vi "Read Port.vi"(8 "error in (no error)":errorcluster, 11 "RS232 to GPIB ConvBox in":refnum<class "RS232 to GPIB ConvBox.lvclass">) -> (0 "error out":errorcluster, 2 "Port":string="Com1", 3 "RS232 to GPIB ConvBox out":refnum<class "RS232 to GPIB ConvBox.lvclass">)   [LabVIEW 2019, in "Protocols.lvlib" / "RS232 to GPIB ConvBox.lvclass"]
uses:
  RS232 to GPIB ConvBox.lvclass
  RS232 to GPIB ConvBox.lvclass/RS232 to GPIB ConvBox.ctl
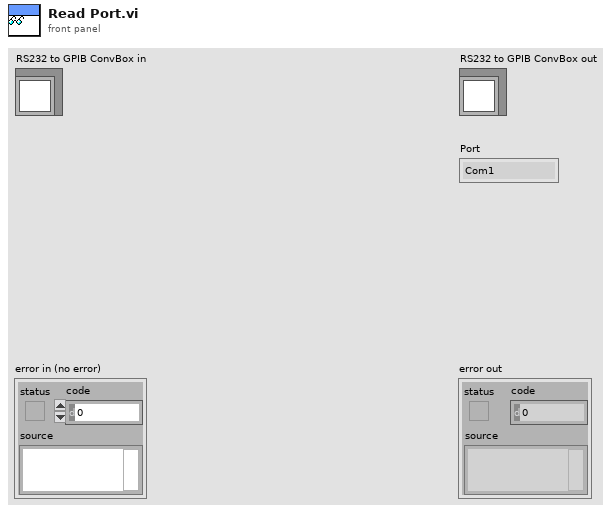
[diagram p1: front panel]
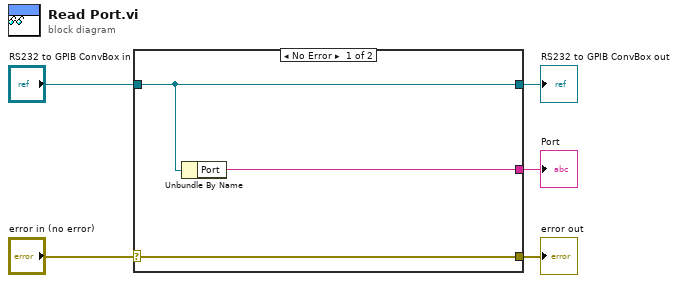
[diagram p0: block diagram]
diagram:
  n1 = case shown="No Error" "error in (no error)" {
    selector: "error in (no error)" -> [w8 w9]
    tunnel: [w8 w9] -> w4
    tunnel: [w7 w10] -> w2
    tunnel: "RS232 to GPIB ConvBox in" -> [w7 w10]
    tunnel: [w6 _] -> w1
    frame No Error {
      n2 = Unbundle By Name(w7) -> ("Port"=w6:string)
    }
    frame Error {
    }
  }
  "error out" <- w4
  "RS232 to GPIB ConvBox out" <- w2
  "Port" <- w1
